vi "Convert Log Entry.vi"(10 "Log Data":T1={"Time"=timestamp(0 s since 1904-01-01), "Level"=enum."INFO", "Logger"="", "Message"="", "Arguments"=[]} {"Time" format="%<%x %.3X>T"}, 11 "Log Sink in":refnum<class "Log Sinks.lvclass">) -> (2 "Log Entry":string)   [LabVIEW 2019, in "TSC Event Logger.lvlib" / "Log Sinks.lvclass"]
uses:
  Log Sinks.lvclass
  Log Data.ctl
  Log/Event Level.ctl
  Log Sinks.lvclass/Log Sinks.ctl
  Layouts/Layout.lvclass
  TSC Event Logger.lvlib
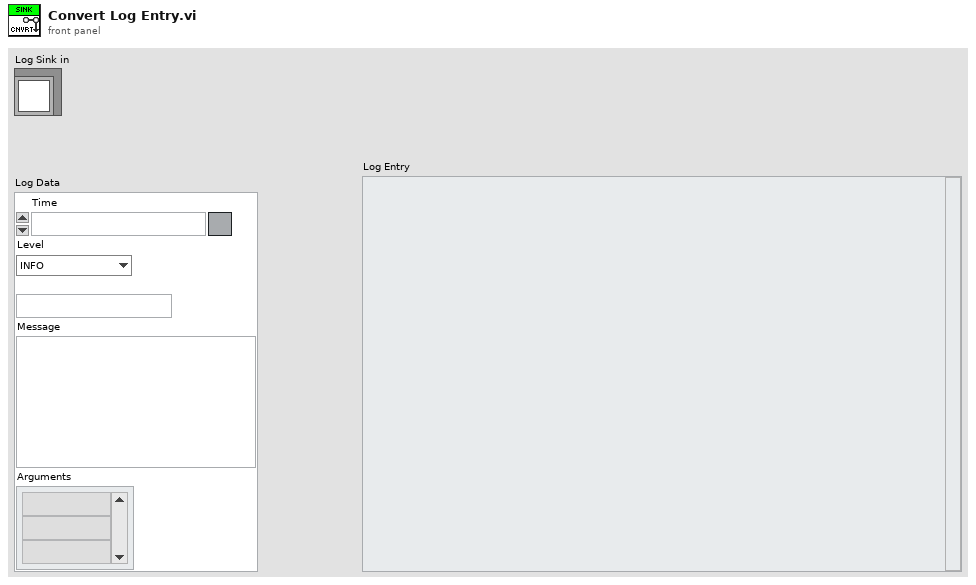
[diagram p1: front panel]
types:
  T1 = typedef "TSC Event Logger.lvlib/Log Data.ctl" = cluster{"Time":timestamp, "Level":T2, "Logger":string, "Message":string, "Arguments":string[]}
  T2 = typedef "TSC Event Logger.lvlib/Event Level.ctl" = enum16{"OFF", "TRACE", "DEBUG", "INFO", "WARN", "ERROR", "FATAL"}
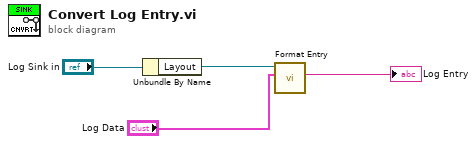
[diagram p0: block diagram]
diagram:
  n1 = Unbundle By Name("Log Sink in") -> ("Layout"=w4:refnum<class "Layout.lvclass">)
  n2 = call-dynamic "Format Entry.vi"("Log Data"="Log Data", "Layout in"=w4) -> ("Log Entry"=→"Log Entry":string)  [unwired: 7 in, 2 out]
